vi "Read Multi Numeric as SGL.vi"(8 "error in (no error)":errorcluster, 9 "Type":sgl[](array[numeric]), 10 "Tag":string[](array[string]), 11 "Var Bus in":refnum<class "Omni_Bus.lvclass">) -> (0 "error out":errorcluster, 2 "Array":sgl[](array[numeric]), 3 "Var Bus out":refnum<class "Omni_Bus.lvclass">)   [LabVIEW 2021, in "Omni_Bus.lvclass"]
uses:
  Omni_Bus.lvclass
  Omni_Bus.lvclass/Omni_Bus.ctl
  <vilib>/TSA/Abstract Data Classes/Abs_Types/Numeric/Abs_Numeric.lvclass
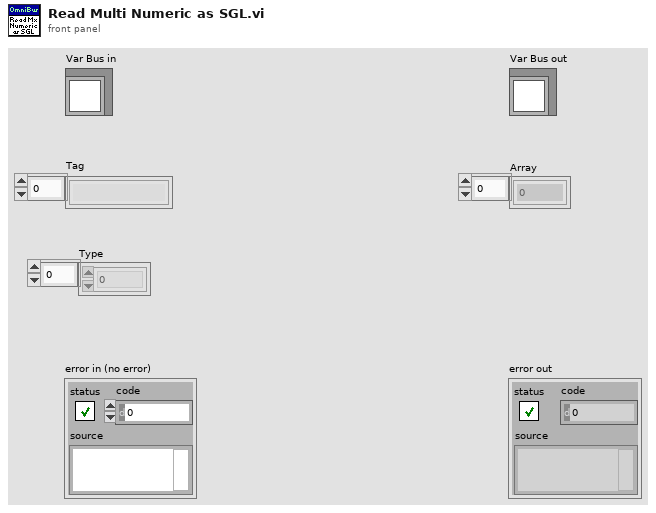
[diagram p1: front panel]
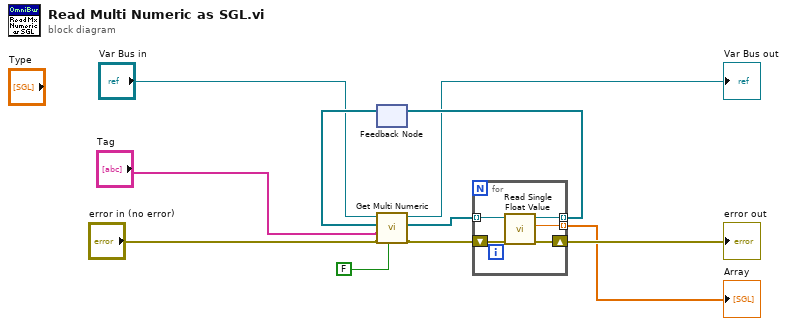
[diagram p0: block diagram]
diagram:
  n1 = feedback #1() -> (w4:refnum<class "Abs_Numeric.lvclass">[])  [unwired: 1 in]
  n2 = call-dynamic "Get Multi Numeric.vi"("Write?"=FALSE, "error in (no error)"="error in (no error)", "Tag"="Tag", "Value Type"=w4, "Var Bus in"="Var Bus in") -> ("error out"=w8:errorcluster, "Value Out"=w7:refnum<class "Abs_Numeric.lvclass">[], "Var Bus out"=→"Var Bus out":refnum<class "Omni_Bus.lvclass">)  [unwired: 4 in]
  n3 = for {
    tunnel: [w15] -> w10 mode=indexing
    tunnel: [w14] -> w9 mode=indexing
    tunnel: w7 -> [w12] mode=indexing
    shift-right: [w16] -> w11
    shift-left: w8 -> [w13]
    n4 = call-dynamic "Read Single Float Value.vi"("error in (no error)"=w13, "Numeric in"=w12) -> ("error out"=w16:errorcluster, "Float"=w15:sgl, "Numeric out"=w14:refnum<class "Abs_Numeric.lvclass">)  [unwired: 7 in]
  }
  "error out" <- w11
  "Array" <- w10
  n5 = feedback-in #1(w9) -> ()
